vi "BarChart2.vi"(9 "Array 3":u8[](array[numeric]), 10 "Array 2":u8[](array[numeric]), 11 "Array":u8[](array[numeric])) -> (3 "XY Graph":cluster{i32[], i32[]}(graph))   [LabVIEW 2014]
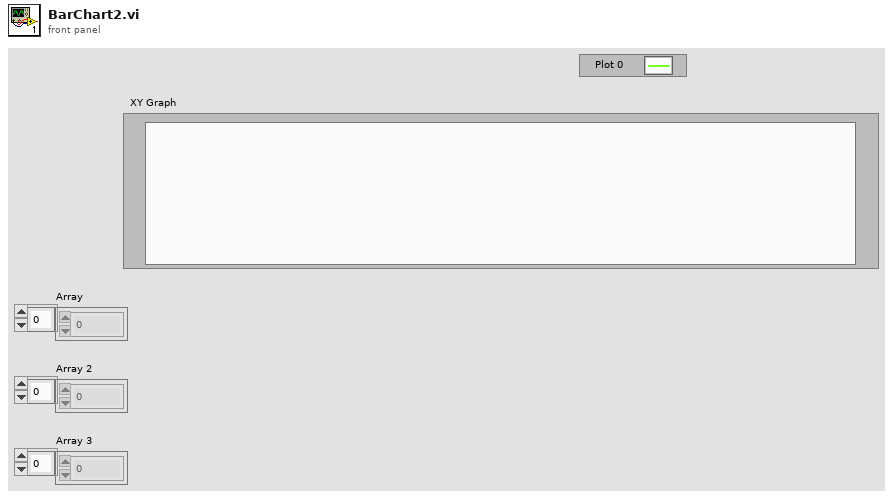
[diagram p1: front panel]
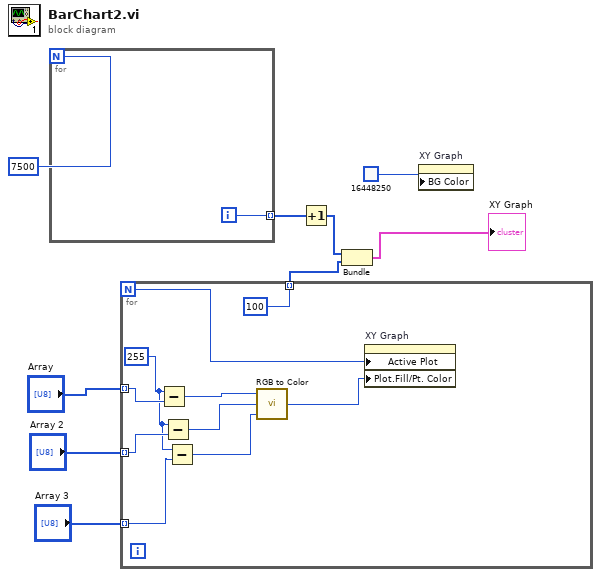
[diagram p0: block diagram]
diagram:
  n1 = for {
    N: 7500 -> [_]
    tunnel: [w10] -> w7 mode=indexing
    i -> [w10]
  }
  n2 = for {
    N -> [w12]
    tunnel: "Array" -> [w18] mode=indexing
    tunnel: "Array 3" -> [w16] mode=indexing
    tunnel: "Array 2" -> [w17] mode=indexing
    tunnel: [100] -> w1 mode=indexing
    w15 = u8 255
    n3 = Subtract(x=w15, y=w18) -> (x-y=w19:u8)
    n4 = Subtract(x=w15, y=w17) -> (x-y=w14:u8)
    n5 = Subtract(x=w15, y=w16) -> (x-y=w13:u8)
    n6 = call <vilib>:"RGB to Color.vi"("B"=w13, "G"=w14, "R"=w19) -> ("Color"=w11:u32)
    n7 = property on="XY Graph" class="XYGraph (strict)"("Active Plot"=w12, "Plot.Fill/Pt. Color"=w11) -> ()  [unwired: 2 in, 2 out]
  }
  n8 = Increment(x=w7) -> (x+1=w6:i32[])
  n9 = Bundle(w6, w1) -> (→"XY Graph":cluster{i32[], i32[]})  [unwired: 1 in]
  n10 = property on="XY Graph" class="XYGraph (strict)"("BG Color"=u32 16448250) -> ()  [unwired: 2 in, 2 out]
